vi "SR865A.vi"(11 "Parameter (1: X)":u16(ring)=1 items=["X"=0, "Y"=1, "R"=2, "Theta"=3, "Channel 1"=8, "Channel 2"=9, "Aux In 1"=12]) -> (3 "data":dbl=-5.2190927136e-07 format="%#_13g")   [LabVIEW 2014]
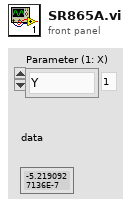
[diagram p1: front panel]
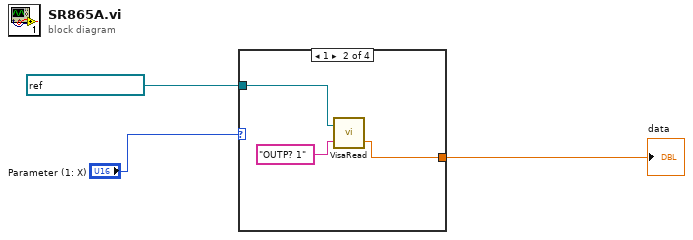
[diagram p0: block diagram]
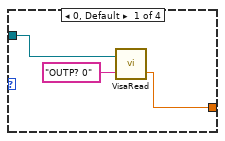
[diagram p2: hidden frame]
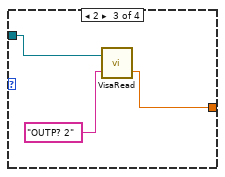
[diagram p3: hidden frame]
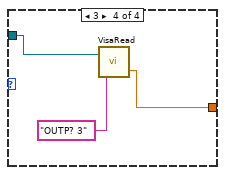
[diagram p4: hidden frame]
diagram:
  n1 = case shown="1" "Parameter (1: X)" {
    tunnel: refnum<visa-resource-name> "GPIB0::7::INSTR" ("VISA资源名称") -> [w6 w9 w12 w15]
    tunnel: [w4 w7 w10 w13] -> w1
    frame 0, Default {
      n2 = call "VisaRead.vi"("command"="OUTP? 0", "VISA资源名称"=w6) -> ("data"=w4:dbl)  [unwired: 1 out]
    }
    frame 1 {
      n3 = call "VisaRead.vi"("command"="OUTP? 1", "VISA资源名称"=w9) -> ("data"=w7:dbl)  [unwired: 1 out]
    }
    frame 2 {
      n4 = call "VisaRead.vi"("command"="OUTP? 2", "VISA资源名称"=w12) -> ("data"=w10:dbl)  [unwired: 1 out]
    }
    frame 3 {
      n5 = call "VisaRead.vi"("command"="OUTP? 3", "VISA资源名称"=w15) -> ("data"=w13:dbl)  [unwired: 1 out]
    }
  }
  "data" <- w1
